vi "Insert PossibleReason In Error.vi"(2 "Possible Reason":string, 4 "error in":errorcluster, 6 "Append (T)":bool=TRUE, 7 "Bold (F)":bool) -> (1 "error out":errorcluster)   [LabVIEW 2025, in "XNode Support.lvlib"]
uses:
  XNode Support.lvlib
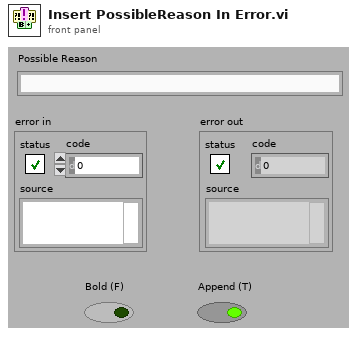
[diagram p1: front panel]
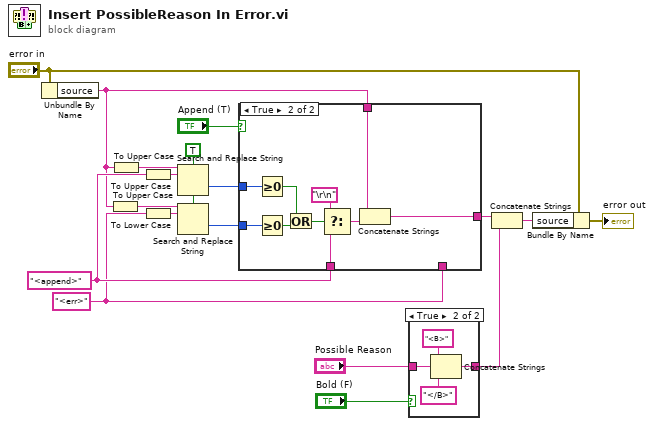
[diagram p0: block diagram]
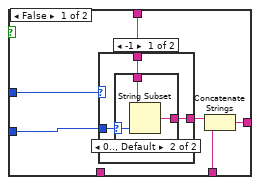
[diagram p2: hidden frame]
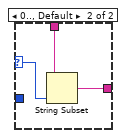
[diagram p4: hidden frame]
diagram:
  w5 = TRUE ("ignore case? (F)")
  w6 = "<err>" ("search string")
  w10 = "<append>" ("search string")
  n1 = Unbundle By Name("error in") -> ("source"=w8:string)
  n2 = To Upper Case(1:w8) -> (0:w2:string)
  n3 = To Upper Case(1:w8) -> (0:w3:string)
  n4 = To Upper Case(1:w10) -> (0:w4:string)
  n5 = To Lower Case(string=w6) -> (all lower case string=w1:string)
  n6 = Search and Replace String(case sensitive?=w5, input string=w3, search string=w4) -> (offset past replacement=w9:i32)  [unwired: 5 in, 3 out]
  n7 = Search and Replace String(case sensitive?=w5, input string=w2, search string=w1) -> (offset past replacement=w7:i32)  [unwired: 5 in, 3 out]
  n8 = case shown="True" "Append (T)" {
    tunnel: [w21 w42] -> w15
    tunnel: w8 -> [w23 w43]
    tunnel: w10 -> [_ w41]
    tunnel: w9 -> [w24 w40]
    tunnel: w7 -> [w20 w38]
    tunnel: w6 -> [w19 _]
    frame False {
      n9 = case shown="-1" w24 {
        selector: w24 -> [_ w33]
        tunnel: w23 -> [w27 w34]
        tunnel: [w26 w32] -> w22
        tunnel: w20 -> [w25 _]
        frame -1 {
          n10 = case shown="0.., Default" w25 {
            selector: w25 -> [_ w30]
            tunnel: w27 -> [w28 w31]
            tunnel: [w28 w29] -> w26
            frame -1 {
            }
            frame 0.., Default {
              n11 = String Subset(string=w31, length (rest)=w30) -> (substring=w29:string)  [unwired: 1 in]
            }
          }
        }
        frame 0.., Default {
          n12 = String Subset(string=w34, length (rest)=w33) -> (substring=w32:string)  [unwired: 1 in]
        }
      }
      n13 = Concatenate Strings(w22, w19) -> (w21:string)
    }
    frame True {
      n14 = Greater Or Equal To 0?(x=w40) -> (x >= 0?=w35:bool)
      n15 = Greater Or Equal To 0?(x=w38) -> (x >= 0?=w37:bool)
      n16 = Or(x=w35, y=w37) -> (x .or. y?=w36:bool)
      n17 = Select(t="\r\n", s=w36, f=w41) -> (s? t:f=w39:string)
      n18 = Concatenate Strings(w43, w39) -> (w42:string)
    }
  }
  n19 = case shown="True" "Bold (F)" {
    tunnel: "Possible Reason" -> [w45 w49]
    tunnel: [w45 w48] -> w12
    frame False {
    }
    frame True {
      n20 = Concatenate Strings("<B>" ("string"), w49, "</B>" ("string")) -> (w48:string)
    }
  }
  n21 = Concatenate Strings(w15, w12) -> (w16:string)
  n22 = Bundle By Name(cluster="error in", "source"=w16) -> (→"error out":errorcluster)
